vi "FRCts20_WebMethods_Events_PUT.vi"(7 "httpRequestID":u32, 11 "team_tickname":string) -> ()   [LabVIEW 2013, in "FRCts20_WebMethods.lvlib"]
doc: "<B>PUT</B> on the specified <B>competition</B> resource\n\n<B>Required Data : </B>\n<Competition>\n <Start_Date><B>YYYY-MM-DD</B></Start_Date>\n <Duration><B>uInt</B></Duration>\n</Competition>\n\nhttp://<server address>:<port>/FRCts/competition/<B>competition</B>\n\n{requires authentication}"
uses:
  FRCts20_WebMethods.lvlib
  <vilib>/wsapi/NI_WebServices.lvlib
  Backend/source/VI Source/FRCts20_Backend_API/FRCts20_Backend_API.lvlib
  Backend/source/VI Source/FRCts20_Backend_API/FRCts20_Backend_API_Event.vi
  Backend/source/VI Source/FRCts20_Backend_API/FRCts20_Backend_API_Command_Event.ctl
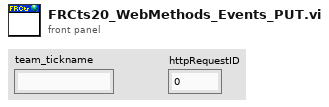
[diagram p1: front panel]
types:
  T1 = typedef "FRCts20_Backend_API.lvlib/FRCts20_Backend_API_Command_Event.ctl" = string
  T2 = typedef "FRCts20_WebMethods.lvlib/FRCts20_WebMethods_ctl_singleEvent.ctl" = cluster{"Team":T3[], "Issue Count":i32, "Location":string, "Start Date ":timestamp}
  T3 = typedef "FRCts20_WebMethods.lvlib/FRCts20_WebMethods_ctl_teamIdentifier.ctl" = cluster{"Team Nickname":string, "Team Number ":u32, "UniqueId":u32}
  T4 = typedef "FRCts20_WebMethods.lvlib/FRCts20_WebMethods_ctl_returntype.ctl" = string
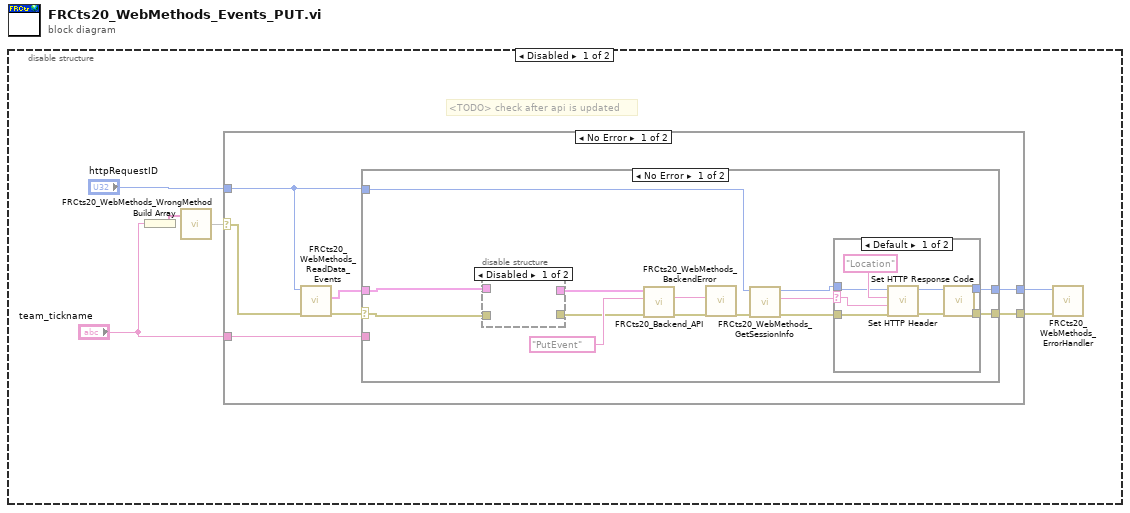
[diagram p0: block diagram]
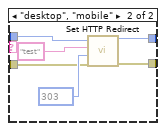
[diagram p3: hidden frame]
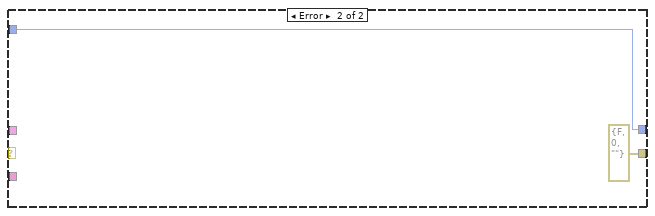
[diagram p4: hidden frame]
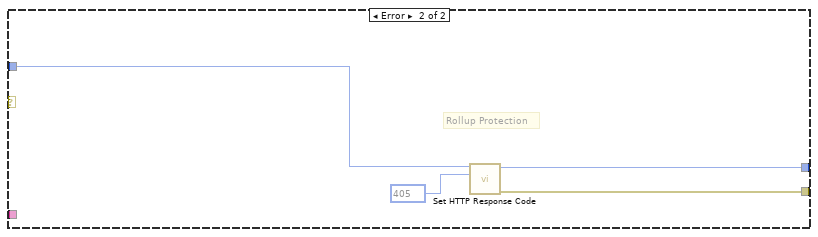
[diagram p5: hidden frame]
diagram:
  n1 = disable-structure shown="Disabled" {
    frame Disabled {
      # "<TODO> check after api is updated"
      n2 = Build Array("team_tickname") -> (w4:string[])
      n3 = call "FRCts20_WebMethods_WrongMethod.vi"(4:w4) -> (1:w5)  [unwired: 3 in, 1 out]
      n4 = case shown="No Error" w5 {
        selector: w5 -> [w9 _]
        tunnel: "httpRequestID" -> [w10 w46]
        tunnel: [w13 w45] -> w3
        tunnel: [w12 w44] -> w2
        tunnel: "team_tickname" -> [w11 _]
        frame No Error {
          n5 = call "FRCts20_WebMethods_ReadData_Events.vi"("error in (no error)"=w9, "httpRequestID"=w10) -> ("error out"=w8:errorcluster, "Single Event out"=w7:T2)  [unwired: 7 in, 1 out]
          n6 = case shown="No Error" w8 {
            selector: w8 -> [w16 _]
            tunnel: w10 -> [w22 w43]
            tunnel: [w24 errorcluster {"status"=FALSE, "code"=0, "source"=""} ("error out")] -> w13
            tunnel: [w18 w43] -> w12
            tunnel: w11 -> [_ _]
            tunnel: w7 -> [w17 _]
            frame No Error {
              n7 = disable-structure shown="Disabled" {
                disable-tunnel: w17 -> [_ _]
                disable-tunnel: w16 -> [_ _]
                disable-tunnel: [_ _] -> w15
                disable-tunnel: [_ _] -> w14
                frame Disabled {
                }
                frame Enabled {
                }
              }
              n8 = call-poly "FRCts20_Backend_API.vi"("error in (no error)"=w15, "Command"=T1 "PutEvent", "Event In"=w14) -> ("error out"=w26:errorcluster, "Status"=w25:string)  [unwired: 6 in, 1 out]
              n9 = call "FRCts20_WebMethods_BackendError.vi"("error in (no error)"=w26, "Status"=w25) -> ("error out"=w23:errorcluster)  [unwired: 8 in, 1 out]
              n10 = call "FRCts20_WebMethods_GetSessionInfo.vi"("error in"=w23, "httpRequestID"=w22) -> ("error out"=w19:errorcluster, "Return Type"=w21:T4, "httpRequestID out"=w20:u32)  [unwired: 7 in]
              n11 = case shown="Default" w21 {
                selector: w21 -> [w28 _]
                tunnel: [w34 w41] -> w24
                tunnel: [w31 w40] -> w18
                tunnel: w20 -> [w30 w38]
                tunnel: w19 -> [w29 w37]
                frame Default {
                  n12 = call <vilib>:"Set HTTP Header.vi"("error in (no error)"=w29, "header value"=w28, "header"="Location", "httpRequestID"=w30) -> ("error out"=w33:errorcluster, "httpRequestID out"=w32:u32)  [unwired: 6 in]
                  n13 = call <vilib>:"Set HTTP Response Code.vi"("error in (no error)"=w33, "httpRequestID"=w32) -> ("error out"=w34:errorcluster, "httpRequestID out"=w31:u32)  [unwired: 8 in]
                }
                frame "desktop", "mobile" {
                  w39 = 303 items=["100"=100, "101"=101, "200"=200, "201"=201, "202"=202, "203"=203, "204"=204, "205"=205, "206"=206, "300"=300, "301"=301, "302"=302, "303"=303, "304"=304, "305"=305, "306"=306, "307"=307, "400"=400, "401"=401, "402"=402, "403"=403, "404"=404, "405"=405, "406"=406, "407"=407, "408"=408, "409"=409, "410"=410, "411"=411, "412"=412, "413"=413, "414"=414, "415"=415, "416"=416, "417"=417, "500"=500, "501"=501, "502"=502, "503"=503, "504"=504, "505"=505] ("response code (307)")
                  n14 = call <vilib>:"Set HTTP Redirect.vi"("error in (no error)"=w37, "response code (307)"=w39, "redirect URL"="test", "httpRequestID"=w38) -> ("error out"=w41:errorcluster, "httpRequestID out"=w40:u32)  [unwired: 6 in]
                }
              }
            }
            frame Error {
            }
          }
        }
        frame Error {
          w47 = 405 items=["100"=100, "101"=101, "200"=200, "201"=201, "202"=202, "203"=203, "204"=204, "205"=205, "206"=206, "300"=300, "301"=301, "302"=302, "303"=303, "304"=304, "305"=305, "306"=306, "307"=307, "400"=400, "401"=401, "402"=402, "403"=403, "404"=404, "405"=405, "406"=406, "407"=407, "408"=408, "409"=409, "410"=410, "411"=411, "412"=412, "413"=413, "414"=414, "415"=415, "416"=416, "417"=417, "500"=500, "501"=501, "502"=502, "503"=503, "504"=504, "505"=505] ("response code (200)")
          # "Rollup Protection"
          n15 = call <vilib>:"Set HTTP Response Code.vi"("response code (200)"=w47, "httpRequestID"=w46) -> ("error out"=w45:errorcluster, "httpRequestID out"=w44:u32)  [unwired: 8 in]
        }
      }
      n16 = call "FRCts20_WebMethods_ErrorHandler.vi"("error in"=w3, "httpRequestID"=w2) -> ()  [unwired: 9 in, 1 out]
    }
    frame Enabled {
    }
  }
